vi "Main.vi"() -> ()   [LabVIEW 2021]
uses:
  <vilib>/Utility/file.llb/Read Delimited Spreadsheet (string).vi
panel:
  out ".not. x?":bool
  out "Final Result":string
  out "?":string[][](array[string])
  out "?":path
  in  "Path":path
  out "concatenated string":string
  out "Lucky Number":u8
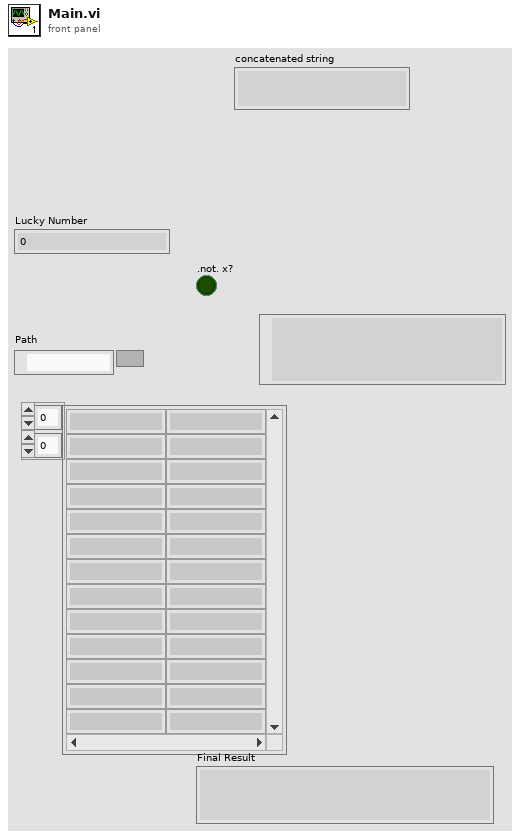
[diagram p1: front panel]
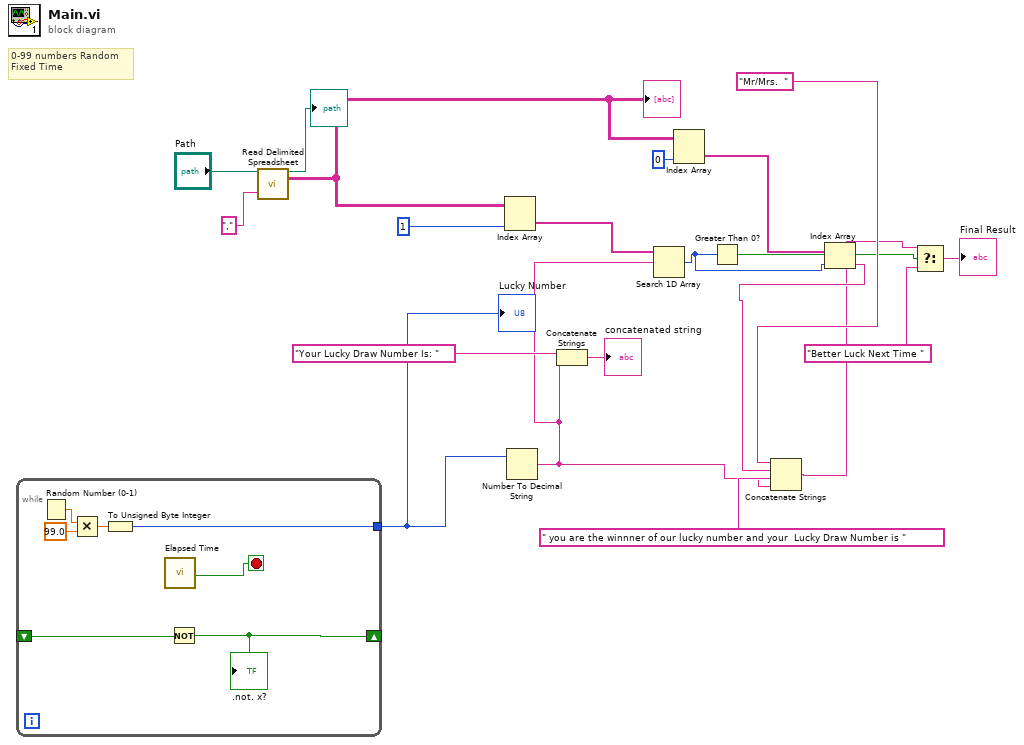
[diagram p0: block diagram]
diagram:
  # "0-99 numbers Random\nFixed Time"
  n1 = while {
    tunnel: [w24] -> w20
    shift-right: [w21] -> _
    shift-left: _ -> [w22]
    stop <- w23 stop-if-true
    n2 = Random Number (0-1)() -> (number: 0 to 1=w27:dbl)
    n3 = Multiply(x=w27, y=99.0) -> (x*y=w25:dbl)
    n4 = To Unsigned Byte Integer(number=w25) -> (unsigned 8bit integer=w24:u8)
    n5 = call "Elapsed Time"() -> ("Time has Elapsed"=w23:bool)  [unwired: 12 in, 7 out]
    n6 = Not(x=w22) -> (.not. x?=w21:bool)
    ".not. x?" <- w21
  }
  "Lucky Number" <- w20
  n7 = call-poly <vilib>:"Read Delimited Spreadsheet.vi"("file path (dialog if empty)"="Path", "delimiter (\\t)"="," ("delimiter (\\t)")) -> ("new file path (Not A Path if cancelled)"=→"?":path, "all rows"=w12:string[][])  [unwired: 8 in, 4 out]
  "?" <- w12
  n8 = Index Array(array=w12, index (col)=1 ("disabled index (col)")) -> (element=w13:string[])  [unwired: 1 in]
  n9 = Number To Decimal String(number=w20) -> (decimal integer string=w7:string)  [unwired: 1 in]
  n10 = Concatenate Strings("Your Lucky Draw Number Is: ", w7) -> (→"concatenated string":string)
  n11 = Search 1D Array(1D array=w13, element=w7) -> (index of element=w5:i32)  [unwired: 1 in]
  n12 = Index Array(array=w12, index (col)=0 ("disabled index (col)")) -> (element=w10:string[])  [unwired: 1 in]
  n13 = Greater Than 0?(x=w5) -> (x > 0?=w4:bool)
  n14 = Index Array(array=w10, index=w5) -> (element=w6:string)
  n15 = Concatenate Strings("Mr/Mrs.  ", w6, " you are the winnner of our lucky number and your  Lucky Draw Number is ", w7) -> (w3:string)
  n16 = Select(t=w3, s=w4, f="Better Luck Next Time ") -> (s? t:f=→"Final Result":string)
